vi "Interface.RT FIFO.Delete.vi"   [LabVIEW 2017, in "DSF Core.lvlib" / "Interface.lvclass"]
uses:
  Interface.lvclass
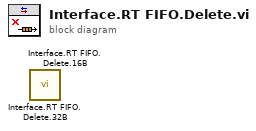
[diagram p0: block diagram]
diagram:
  n1 = call "Interface.RT FIFO.Delete.32B.vi"() -> ()  [unwired: 11 in, 1 out]
  n2 = call "Interface.RT FIFO.Delete.16B.vi"() -> ()  [unwired: 11 in, 1 out]
